vi "Main.vi"() -> ()   [LabVIEW 2017]
uses:
  <vilib>/Analysis/baseanly.llb/Mean (DBL).vi
  <vilib>/Analysis/NI_AALBase.lvlib
panel:
  in  "Save Raw Spectrometer Data":bool=TRUE
  out "Spectrometer Data":T1={[750.0, 800.0], "mean"=-22.554463094146342, array[2540 elements], array[2540 elements], "Color Temperatures"=[[-3182.0998200450113], [-4677.963743364752], [-7826.4943596651665]]}
  out "Voltage Average":dbl
  in  "Wait time (ms)":i32=250
  out "Motor Cluster":cluster{"Motor Relative":dbl[]}={"Motor Relative"=[0.0900112499774972, 0.0, 0.0, 0.0]}
  in  "WL2":dbl=800.0 format="%#_13g"
  in  "WL1":dbl=750.0 format="%#_13g"
  in  "Y axis":T2(ring)=enum."Spectrometer intensity"
  in  "Clear data":bool
  in  "Vi Selection":bool[](array[boolean])=[FALSE, TRUE, TRUE, TRUE, FALSE]
  in  "base path":path=path "E:/Materials Testing"
  in  "Filename":string="Run1"
  in  "stop":bool
  out "XY Graph":cluster{"magnitude":dbl[], dbl[]}(graph)
  in  "X axis":T3(ring)=enum."Spectrometer Wavelength"
  # "Power Meter"
  # "Spectrometer"
  # "Sensors"
  # "Motor"
  # "Keithley"
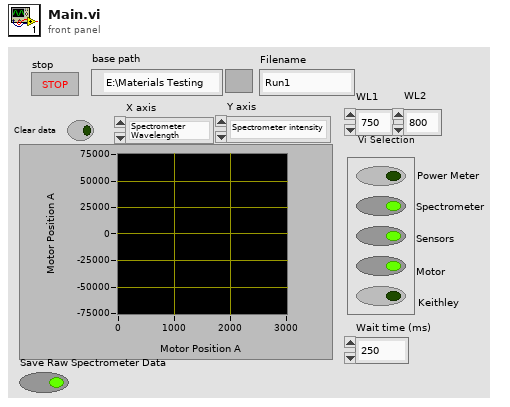
[diagram p1: front panel]
types:
  T1 = cluster{dbl[], "mean":dbl, dbl[], dbl[], "Color Temperatures":dbl[][]}
  T2 = enum16{"Motor Position A", "Motor Position B", "Motor Position C", "Motor Position D", "Spectrometer Region Avg.", "Keithley Voltage", "Spectrometer intensity", "Color Temp 2 -3", "Color Temp 1-3", "Color Temp 1-2"}
  T3 = enum16{"Time", "Motor Position A", "Motor Position B", "Motor Position C", "Motor Position D", "Spectrometer Wavelength"}
  T4 = enum16{"PowerMeter", "Spectrometer", "Sensors", "Motor", "Keithley"}
  T5 = enum32{"Invalid", "Standard", "Closed", "Hidden", "Minimized", "Maximized"}
  T6 = cluster{"output cluster 2":cluster{"Value:":dbl[], timestamp[], string[][]}, "output cluster 3":cluster{"Value:":dbl[], timestamp[], string[][]}}
  T7 = cluster{"Temperature Data":cluster{"Bandwidth":i32[], "Bandwidth labels":string[], "Color Temperatures":dbl[][], "Wavelength labels":string[], "seconds since 1Jan1904":timestamp}, "Vis Data":cluster{cluster{"visible wl array":dbl[], dbl[]}, cluster{"Vis or NIR":string, "Multiplexer Response":string, "Wavelength Difference Vis (nm)":dbl, "Vis Integration Time (ms)":u32, "Normalization path":path, "Vis background wave":cluster{dbl[], dbl[]}}}, "NIR Data":cluster{cluster{"NIR wl array":dbl[], dbl[]}, cluster{"Vis or NIR":string, "Multiplexer Response":string, "NIR Integration Time (ms)":u32, "Wavelength Difference NIR (nm) ":dbl, "Normalization path":path, "NIR background wave":cluster{dbl[], dbl[]}}}}
  T8 = cluster{dynamicdata, dynamicdata, dynamicdata, "Dynamic Data Type":dynamicdata}
  T9 = cluster{"Motor Relative":dbl[], "Motor absolute":dbl[], "Motor zero":dbl[], "Time between steps":dbl, "Conversion (steps/mm)":dbl[], "Distance  (mm)":dbl[], "run number":i32, "Number of steps":i32}
  T10 = cluster{"mean":dbl, "seconds since 1Jan1904":timestamp}
  T11 = enum32{"Bad", "Idle", "Run top level", "Running"}
  T12 = cluster{"VI out":refnum<vi>, "error out":errorcluster, refnum<vi>, enum16{"PowerMeter", "Spectrometer", "Sensors", "Motor", "Keithley"}, "Run Power meter":bool}
  T13 = enum16{"open", "open or create", "create or replace", "create", "open (read-only)"}
  T14 = cluster{"Bandwidth":i32[], "Bandwidth labels":string[], "Color Temperatures":dbl[][], "Wavelength labels":string[], "seconds since 1Jan1904":timestamp}
  T15 = cluster{cluster{"visible wl array":dbl[], dbl[]}, cluster{"Vis or NIR":string, "Multiplexer Response":string, "Wavelength Difference Vis (nm)":dbl, "Vis Integration Time (ms)":u32, "Normalization path":path, "Vis background wave":cluster{dbl[], dbl[]}}}
  T16 = cluster{cluster{"NIR wl array":dbl[], dbl[]}, cluster{"Vis or NIR":string, "Multiplexer Response":string, "NIR Integration Time (ms)":u32, "Wavelength Difference NIR (nm) ":dbl, "Normalization path":path, "NIR background wave":cluster{dbl[], dbl[]}}}
  T17 = cluster{"Vis or NIR":string, "Multiplexer Response":string, "NIR Integration Time (ms)":u32, "Wavelength Difference NIR (nm) ":dbl, "Normalization path":path, "NIR background wave":cluster{dbl[], dbl[]}}
  T18 = cluster{"Vis or NIR":string, "Multiplexer Response":string, "Wavelength Difference Vis (nm)":dbl, "Vis Integration Time (ms)":u32, "Normalization path":path, "Vis background wave":cluster{dbl[], dbl[]}}
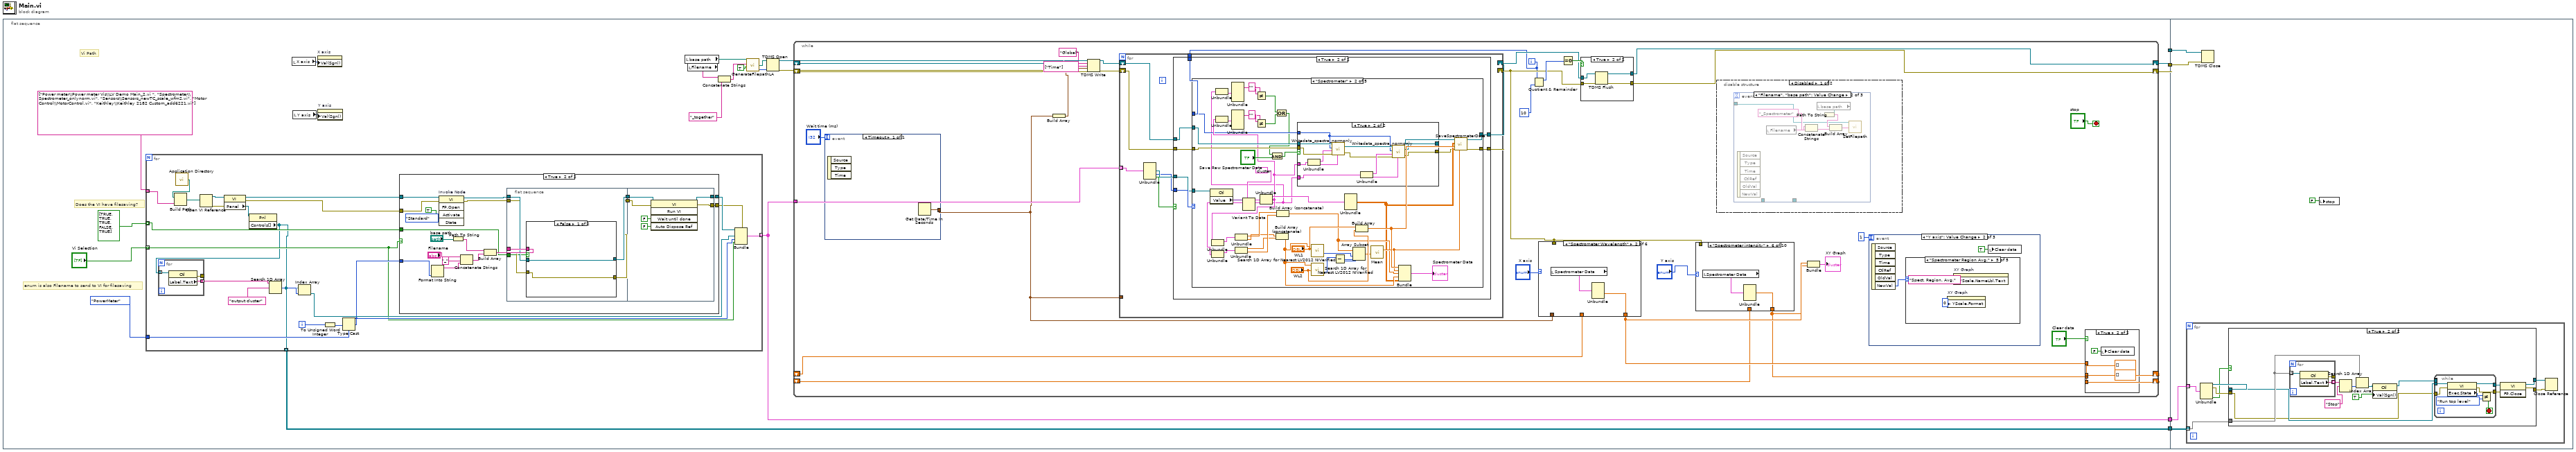
[diagram p0: block diagram]
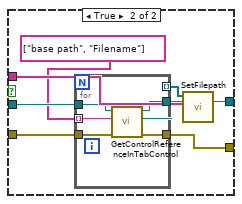
[diagram p3: hidden frame]
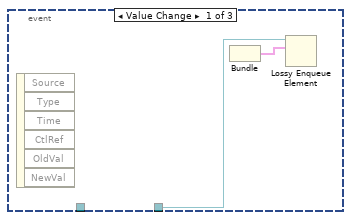
[diagram p5: hidden frame]
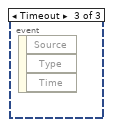
[diagram p6: hidden frame]
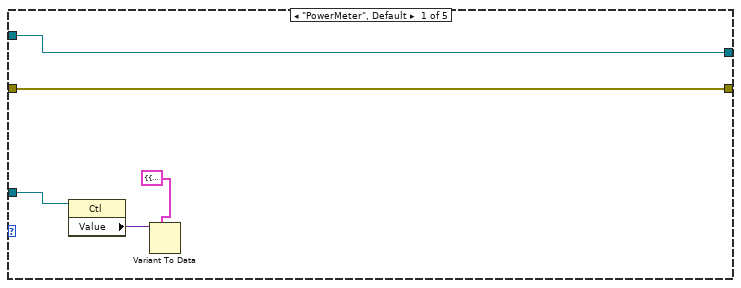
[diagram p9: hidden frame]
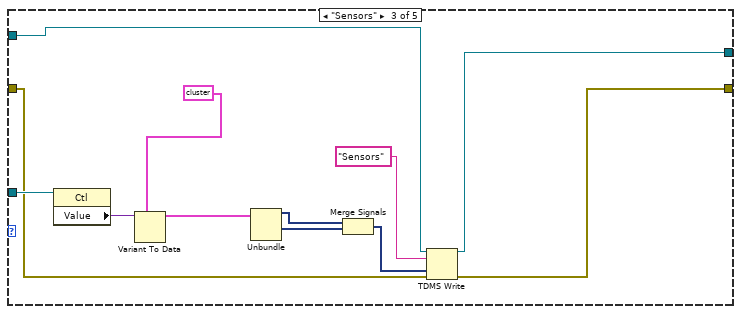
[diagram p11: hidden frame]
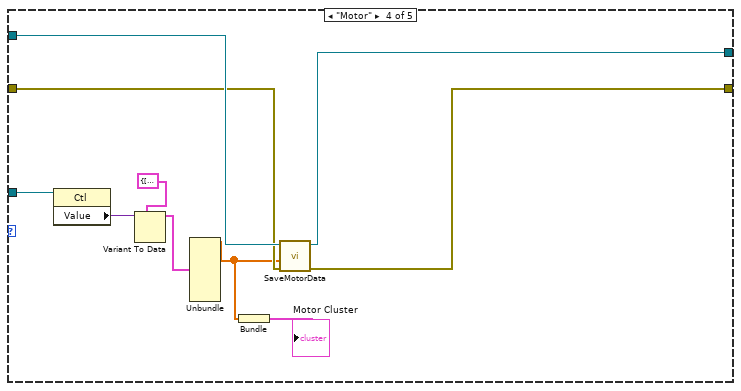
[diagram p12: hidden frame]
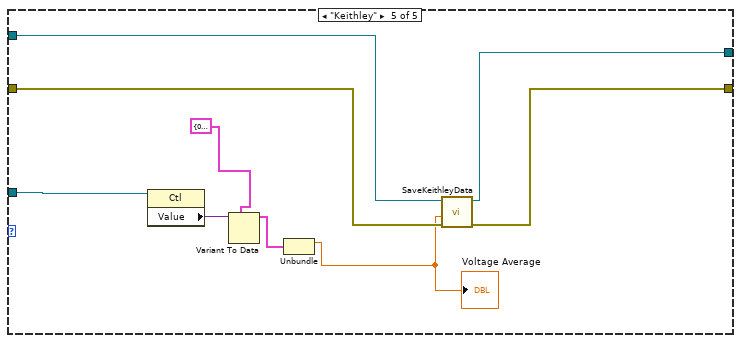
[diagram p13: hidden frame]
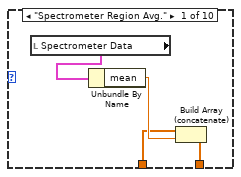
[diagram p15: hidden frame]
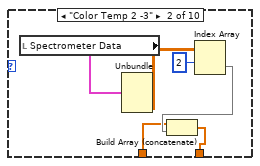
[diagram p16: hidden frame]
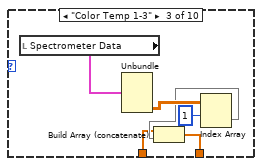
[diagram p17: hidden frame]
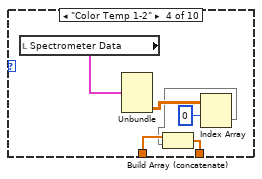
[diagram p18: hidden frame]
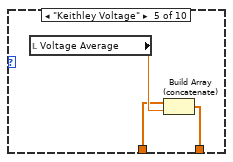
[diagram p19: hidden frame]
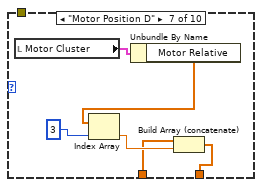
[diagram p20: hidden frame]
diagram:
  n1 = flat-sequence {
    tunnel: [w9] -> w4
    tunnel: [w10] -> w3
    tunnel: [w11] -> w2
    tunnel: [w7] -> w1
    tunnel: w4 -> [w370]
    tunnel: w3 -> [w369]
    tunnel: w2 -> [w368]
    tunnel: w1 -> [w367]
    frame #0 {
      # "Does the VI have filesaving?"
      # "enum is also Filename to send to VI for filesaving"
      # "Vi Path"
      n2 = for {
        tunnel: string[] ["Power meter\\Power meter Vis\\LV Demo Main_2.vi ", "Spectrometer\\Spectrometer_onlynorm.vi", "Sensors\\Sensors_newTC_scale_wfm2.vi", "Motor Control\\MotorControl.vi", "Keithley\\Keithley 2182 Custom_add6221.vi"] ("name or relative path") -> [w45] mode=indexing
        tunnel: bool[] [TRUE, TRUE, TRUE, FALSE, TRUE] ("Vi Selection 2") -> [w26] mode=indexing
        tunnel: T4."PowerMeter" -> [w44]
        tunnel: [w29] -> w11 mode=indexing
        tunnel: "Vi Selection" -> [w25] mode=indexing
        tunnel: [w24] -> w7 mode=indexing
        i -> [w43]
        n3 = call <vilib>:"Application Directory.vi"() -> ("Application Directory"=w38:path)
        n4 = Build Path(base path=w38, name or relative path=w45) -> (appended path=w34:path)
        n5 = Open VI Reference(vi path=w34) -> (vi reference=w36:refnum<vi>, error out=w37:errorcluster)  [unwired: 5 in]
        n6 = property class="VI"(reference=w36, error in=w37) -> (reference out=w41:refnum<vi>, error out=w39:errorcluster, "Panel"=w42:refnum<vi>)
        n7 = property class="Pnl"(reference=w42) -> ("Controls[]"=w24:refnum<vi>[])  [unwired: 1 in, 2 out]
        n8 = for {
          tunnel: w24 -> [w96] mode=indexing
          tunnel: [w95] -> w40 mode=indexing
          tunnel: [w94] -> _
          n9 = property class="Ctl"(reference=w96) -> (error out=w94:errorcluster, "Label.Text"=w95:string)  [unwired: 1 in, 1 out]
        }
        n10 = Search 1D Array(1D array=w40, element="output cluster") -> (index of element=w35:i32)  [unwired: 1 in]
        n11 = Index Array(array=w24, index=w35) -> (element=w28:refnum<vi>)
        n12 = To Unsigned Word Integer(number=w43) -> (unsigned 16bit integer=w30:u16)
        n13 = Type Cast(type=w44, x=w30) -> (*(type *) &x=w27:T4)
        n14 = case shown="True" w25 {
          tunnel: [w47 w59] -> w32
          tunnel: [w46 w58] -> w31
          tunnel: w41 -> [w47 w53]
          tunnel: w39 -> [w46 w52]
          tunnel: w27 -> [_ w49]
          tunnel: w26 -> [_ w48]
          frame False {
          }
          frame True {
            n15 = Format Into String(w49) -> (resulting string=w56:string)  [unwired: 3 in, 1 out]
            n16 = invoke on="Invoke Node" class="VI" method="FP.Open"(reference=w53, error in=w52, "Activate"=TRUE ("Activate?"), "State"=T5."Standard") -> (reference out=w51:refnum<vi>, error out=w50:errorcluster)  [unwired: 1 in, 3 out]
            n17 = Path To String(path="base path") -> (string=w62:string)
            n18 = Concatenate Strings("Filename", "_" ("string"), w56) -> (w63:string)
            n19 = Build Array(w62, w63) -> (w64:string[])
            n20 = flat-sequence {
              tunnel: w50 -> [w70]
              tunnel: w64 -> [w72]
              tunnel: w51 -> [w71]
              tunnel: [w69] -> w66
              tunnel: [w68] -> w65
              tunnel: w48 -> [w67]
              tunnel: w66 -> [w91]
              tunnel: w65 -> [w89]
              tunnel: [w90] -> w59
              tunnel: [w88] -> w58
              frame #0 {
                n21 = case shown="False" w67 {
                  tunnel: w72 -> [_ w81]
                  tunnel: w71 -> [w74 w79]
                  tunnel: w70 -> [w73 w78]
                  tunnel: [w74 w76] -> w69
                  tunnel: [w73 w75] -> w68
                  frame False {
                  }
                  frame True {
                    n22 = for {
                      tunnel: string[] ["base path", "Filename"] -> [w87] mode=indexing
                      tunnel: w79 -> [w86]
                      tunnel: w78 -> [w85]
                      tunnel: [w84] -> w76
                      tunnel: [w83] -> w75
                      tunnel: [w82] -> w80 mode=indexing
                      n23 = call "GetControlReferenceInTabControl.vi"("error in (no error)"=w85, "Control Name"=w87, "VI in"=w86) -> ("error out"=w83:errorcluster, "Ctl Refnum"=w82:refnum<vi>, "VI out"=w84:refnum<vi>)  [unwired: 6 in]
                    }
                    n24 = call "SetFilepath.vi"("Array 2"=w81, "Array"=w80) -> ()  [unwired: 10 in]
                  }
                }
              }
              frame #1 {
                n25 = invoke class="VI" method="Run VI"(reference=w91, error in=w89, "Wait until done"=FALSE ("Wait Until Done"), "Auto Dispose Ref"=FALSE ("Auto Dispose Reference")) -> (reference out=w90:refnum<vi>, error out=w88:errorcluster)  [unwired: 1 in, 3 out]
              }
            }
          }
        }
        n26 = Bundle("VI out"=w32, "error out"=w31, w28, w27, "Run Power meter"=w25) -> (w29:T12)  [unwired: 1 in]
      }
      n27 = local read "X axis"() -> (w6:T3)
      n28 = local read "Y axis"() -> (w5:T2)
      n29 = property on="X axis" class="Enum (strict)"("Val(Sgnl)"=w6) -> ()  [unwired: 2 in, 2 out]
      n30 = property on="Y axis" class="Enum (strict)"("Val(Sgnl)"=w5) -> ()  [unwired: 2 in, 2 out]
      n31 = local read "base path"() -> (w21:path)
      n32 = local read "Filename"() -> (w17:string)
      n33 = Concatenate Strings(w17, "_together" ("string")) -> (w15:string)
      n34 = call "GenerateFilepathLA.vi"("Auto Date folder"=TRUE, "Filename"=w15, "base path"=w21) -> ("operation (0:open)"=w22:T13, "file path"=w20:path)  [unwired: 1 in, 1 out]
      n35 = TDMS Open(10:w22, 11:w20) -> (0:w19:errorcluster, 3:w18:refnum<k34>)  [unwired: 5 in]
      n36 = while {
        shift-right: [w106] -> w10
        shift-left: w18 -> [w115]
        shift-right: [w105] -> w9
        shift-left: w19 -> [w116]
        tunnel: w11 -> [w119]
        shift-right: [w108] -> _
        shift-left: _ -> [w100]
        shift-right: [w109] -> _
        shift-left: _ -> [w98]
        i -> [w97]
        stop <- "stop" stop-if-true
        n37 = event shown="[0] Timeout" {
          selector: _ -> [_]
          dyn-events: _ -> [_]
          timeout: "Wait time (ms)" -> [_]
          tunnel: [w127] -> w103
          event Timeout {
            n38 = event-data() -> ()  [unwired: 1 in, 3 out]
            n39 = Get Date/Time In Seconds() -> (seconds since 1Jan1904=w127:timestamp)
          }
        }
        n40 = Build Array(w103) -> (w114:timestamp[])
        n41 = TDMS Write(0:w115, 5:"Global" ("group name in (Untitled)"), 7:string[] ["Time"] ("channel name(s) in (Untitled)"), 9:w114, 11:w116) -> (4:w111:refnum<k34>, 15:w110:errorcluster)  [unwired: 1 in, 2 out]
        n42 = for {
          tunnel: w119 -> [w152] mode=indexing
          shift-right: [w149] -> w118
          shift-left: w111 -> [w151]
          shift-right: [w148] -> w104
          shift-left: w110 -> [w150]
          tunnel: w103 -> [_]
          tunnel: w97 -> [w144]
          n43 = Unbundle(w152) -> (w147:refnum<vi>, w146:T4, "Run Power meter"=w145:bool)  [unwired: 2 out]
          n44 = case shown="True" w145 {
            tunnel: w146 -> [_ w161]
            tunnel: w147 -> [_ w160]
            tunnel: w151 -> [w154 w159]
            tunnel: w150 -> [w153 w158]
            tunnel: [w154 w157] -> w149
            tunnel: [w153 w156] -> w148
            tunnel: w144 -> [_ w155]
            frame False {
            }
            frame True {
              n45 = case shown="\"Spectrometer\"" w161 {
                tunnel: w160 -> [w165 w209 w236 w246 w253]
                tunnel: w159 -> [w163 w182 w233 w242 w252]
                tunnel: w158 -> [w162 w181 w232 w240 w251]
                tunnel: [w163 w201 w229 w241 w250] -> w157
                tunnel: [w162 w200 w231 w239 w249] -> w156
                tunnel: w155 -> [_ w174 _ _ _]
                frame "PowerMeter", Default {
                  n46 = property class="Ctl"(reference=w165) -> ("Value"=w166:variant)  [unwired: 1 in, 2 out]
                  n47 = Variant To Data(type=T6 {"output cluster 2"={"Value:"=[], [], []}, "output cluster 3"={"Value:"=[], [], []}} ("Power meter Cluster 2"), Variant=w166) -> ()  [unwired: 1 in, 2 out]
                }
                frame "Spectrometer" {
                  n48 = property class="Ctl"(reference=w209) -> ("Value"=w208:variant)  [unwired: 1 in, 2 out]
                  n49 = Variant To Data(type=T7 {"Temperature Data"={"Bandwidth"=[10, 10, 10], "Bandwidth labels"=["Bandwidth 1-2", "Bandwidth 2-3", "Bandwidth 1-3"], "Color Temperatures"=[[879.3311636229715], [-21903.619530261916], [-1063.75969736004]], "Wavelength labels"=["Temp1050-1120", "Temp1050-1230", "Temp1120-1230"], "seconds since 1Jan1904"=timestamp(3594756427.269044 s since 1904-01-01)}, "Vis Data"={{"visible wl array"=array[512 elements], array[512 elements]}, {"Vis or NIR"="NIR", "Multiplexer Response"="-1", "Wavelength Difference Vis (nm)"=50.0, "Vis Integration Time (ms)"=100, "Normalization path"=path "E:/Materials Testing/Calibration/2017-11-09/Multiplexter.tdms", "Vis background wave"={array[512 elements], array[512 elements]}}}, "NIR Data"={{"NIR wl array"=array[2028 elements], array[2028 elements]}, {"Vis or NIR"="Visible", "Multiplexer Response"="-1", "NIR Integration Time (ms)"=100, "Wavelength Difference NIR (nm) "=100.0, "Normalization path"=path "E:/Materials Testing/Calibration/2017-11-09/Multiplexter.tdms", "NIR background wave"={array[2028 elements], array[2028 elements]}}}} ("output cluster"), Variant=w208) -> (data=w197:T7)  [unwired: 1 in, 1 out]
                  n50 = Unbundle(w197) -> ("Temperature Data"=w183:T14, "Vis Data"=w175:T15, "NIR Data"=w170:T16)
                  n51 = Unbundle(w175) -> (w189:cluster{"visible wl array":dbl[], dbl[]})  [unwired: 1 out]
                  n52 = Unbundle(w170) -> (w188:cluster{"NIR wl array":dbl[], dbl[]})  [unwired: 1 out]
                  n53 = Unbundle(w170) -> (w172:T17)  [unwired: 1 out]
                  n54 = Unbundle(w175) -> (w177:T18)  [unwired: 1 out]
                  n55 = Unbundle(w172) -> ("Multiplexer Response"=w173:string)  [unwired: 5 out]
                  n56 = Unbundle(w177) -> ("Multiplexer Response"=w176:string)  [unwired: 5 out]
                  n57 = Unbundle(w188) -> ("NIR wl array"=w184:dbl[], w186:dbl[])
                  n58 = Unbundle(w189) -> ("visible wl array"=w185:dbl[], w187:dbl[])
                  n59 = Not Equal?(x="", y=w173) -> (x != y?=w169:bool)
                  n60 = Not Equal?(x="", y=w176) -> (x != y?=w168:bool)
                  n61 = Or(x=w169, y=w168) -> (x .or. y?=w167:bool)
                  n62 = And(x=w167, y="Save Raw Spectrometer Data") -> (x .and. y?=w178:bool)
                  n63 = Build Array (concatenate)(w185, w184) -> (w196:dbl[])
                  n64 = Build Array (concatenate)(w187, w186) -> (w195:dbl[])
                  n65 = case shown="True" w178 {
                    tunnel: [w211 w214] -> w180
                    tunnel: w182 -> [w211 w224]
                    tunnel: [w210 w213] -> w179
                    tunnel: w181 -> [w210 w223]
                    tunnel: w175 -> [_ w222]
                    tunnel: w170 -> [_ w219]
                    tunnel: w174 -> [_ w212]
                    frame False {
                    }
                    frame True {
                      n66 = Unbundle(w222) -> (w221:cluster{"visible wl array":dbl[], dbl[]}, w220:T18)
                      n67 = call "Writedata_spectra_normonly.vi"("tdms file in"=w224, "Aquisition number"=w212, "Norm Visible Intensity"=w221, "tdms error in"=w223, "Params"=w220) -> ("tdms file out"=w216:refnum<k34>, "tdms error out"=w215:errorcluster)
                      n68 = Unbundle(w219) -> (w218:cluster{"NIR wl array":dbl[], dbl[]}, w217:T17)
                      n69 = call "Writedata_spectra_normonly.vi"("tdms file in"=w216, "Aquisition number"=w212, "Norm Visible Intensity"=w218, "tdms error in"=w215, "Params"=w217) -> ("tdms file out"=w214:refnum<k34>, "tdms error out"=w213:errorcluster)
                    }
                  }
                  n70 = call "Search 1D Array for Nearest LV2012 NIVerified.vi"("desired element"="WL1", "1D Array"=w196) -> ("closest index"=w202:i32)  [unwired: 8 in, 1 out]
                  n71 = call "Search 1D Array for Nearest LV2012 NIVerified.vi"("desired element"="WL2", "1D Array"=w196) -> ("closest index"=w203:i32)  [unwired: 8 in, 1 out]
                  n72 = Subtract(x=w203, y=w202) -> (x-y=w204:i32)
                  n73 = Unbundle(w183) -> ("Color Temperatures"=w191:dbl[][])  [unwired: 4 out]
                  n74 = Array Subset(array=w195, index=w202, length=w204) -> (w205:dbl[])
                  n75 = Build Array("WL1", "WL2") -> (w199:dbl[])
                  n76 = call-poly <vilib>:"Mean.vi"("X"=w205) -> ("mean"=w198:dbl)  [unwired: 1 out]
                  n77 = Bundle(w199, "mean"=w198, w195, w196, "Color Temperatures"=w191) -> (→"Spectrometer Data":T1)  [unwired: 1 in]
                  n78 = call "SaveSpectrometerData.vi"("Average"=w198, "error in (no error)"=w179, "Wavelengths"=w199, "Color Temperatures"=w191, "Refnum in"=w180) -> ("error out"=w200:errorcluster, "Refnum out"=w201:refnum<k34>)  [unwired: 5 in]
                }
                frame "Sensors" {
                  n79 = property class="Ctl"(reference=w236) -> ("Value"=w235:variant)  [unwired: 1 in, 2 out]
                  n80 = Variant To Data(type=T8 {[], [], [], "Dynamic Data Type"=[]} ("output cluster"), Variant=w235) -> (data=w234:T8)  [unwired: 1 in, 1 out]
                  n81 = Unbundle(w234) -> (w228:dynamicdata, w227:dynamicdata)  [unwired: 2 out]
                  n82 = Merge Signals(w228, w227) -> (w226:dynamicdata)
                  n83 = TDMS Write(0:w233, 5:"Sensors" ("group name in (Untitled)"), 9:w226, 11:w232) -> (4:w229:refnum<k34>, 15:w231:errorcluster)  [unwired: 2 in, 2 out]
                }
                frame "Motor" {
                  n84 = property class="Ctl"(reference=w246) -> ("Value"=w245:variant)  [unwired: 1 in, 2 out]
                  n85 = Variant To Data(type=T9 {"Motor Relative"=[], "Motor absolute"=[], "Motor zero"=[], "Time between steps"=0.0, "Conversion (steps/mm)"=[], "Distance  (mm)"=[], "run number"=0, "Number of steps"=0} ("output cluster 2"), Variant=w245) -> (data=w244:T9)  [unwired: 1 in, 1 out]
                  n86 = Unbundle(w244) -> ("Motor Relative"=w237:dbl[])  [unwired: 7 out]
                  n87 = Bundle("Motor Relative"=w237) -> (→"Motor Cluster":cluster{"Motor Relative":dbl[]})  [unwired: 1 in]
                  n88 = call "SaveMotorData.vi"("error in (no error)"=w240, "Motor Relative"=w237, "Refnum in"=w242) -> ("error out"=w239:errorcluster, "Refnum out"=w241:refnum<k34>)  [unwired: 7 in]
                }
                frame "Keithley" {
                  n89 = property class="Ctl"(reference=w253) -> ("Value"=w255:variant)  [unwired: 1 in, 2 out]
                  n90 = Variant To Data(type=T10 {"mean"=0.0, "seconds since 1Jan1904"=timestamp(0 s since 1904-01-01)} ("output cluster 2"), Variant=w255) -> (data=w254:T10)  [unwired: 1 in, 1 out]
                  n91 = Unbundle(w254) -> ("mean"=w247:dbl)  [unwired: 1 out]
                  "Voltage Average" <- w247
                  n92 = call "SaveKeithleyData.vi"("error in (no error)"=w251, "Voltage average"=w247, "Refnum in"=w252) -> ("error out"=w249:errorcluster, "Refnum out"=w250:refnum<k34>)  [unwired: 7 in]
                }
              }
            }
          }
        }
        n93 = Quotient & Remainder(x=w97, y=10) -> (x-y*floor(x/y)=w120:i32)  [unwired: 1 out]
        n94 = case shown="\"Spectrometer Wavelength\"" "X axis" {
          tunnel: w103 -> [w316 _ _ _ _ _]
          tunnel: w104 -> [_ _ _ _ _ _]
          tunnel: [w314 w317 w319 w326 w332 w337] -> w101
          tunnel: w100 -> [w313 _ w320 w325 w331 w338]
          frame "Time" {
            n95 = To Double Precision Float(number=w316) -> (double precision float=w315:dbl)
            n96 = Build Array (concatenate)(w313, w315) -> (w314:dbl[])
          }
          frame "Spectrometer Wavelength" {
            n97 = local read "Spectrometer Data"() -> (w318:T1)
            n98 = Unbundle(w318) -> (w317:dbl[])  [unwired: 4 out]
          }
          frame "Motor Position A" {
            n99 = local read "Motor Cluster"() -> (w324:cluster{"Motor Relative":dbl[]})
            n100 = Unbundle By Name(w324) -> ("Motor Relative"=w323:dbl[])
            n101 = Index Array(array=w323, index=0 ("disabled index (col)")) -> (element=w321:dbl)
            n102 = Build Array (concatenate)(w320, w321) -> (w319:dbl[])
          }
          frame "Motor Position B" {
            n103 = local read "Motor Cluster"() -> (w330:cluster{"Motor Relative":dbl[]})
            n104 = Unbundle By Name(w330) -> ("Motor Relative"=w329:dbl[])
            n105 = Index Array(array=w329, index=1 ("disabled index (col)")) -> (element=w327:dbl)
            n106 = Build Array (concatenate)(w325, w327) -> (w326:dbl[])
          }
          frame "Motor Position C" {
            n107 = local read "Motor Cluster"() -> (w336:cluster{"Motor Relative":dbl[]})
            n108 = Unbundle By Name(w336) -> ("Motor Relative"=w335:dbl[])
            n109 = Index Array(array=w335, index=2 ("disabled index (col)")) -> (element=w333:dbl)
            n110 = Build Array (concatenate)(w331, w333) -> (w332:dbl[])
          }
          frame "Motor Position D" {
            n111 = local read "Motor Cluster"() -> (w342:cluster{"Motor Relative":dbl[]})
            n112 = Unbundle By Name(w342) -> ("Motor Relative"=w341:dbl[])
            n113 = Index Array(array=w341, index=3 ("disabled index (col)")) -> (element=w339:dbl)
            n114 = Build Array (concatenate)(w338, w339) -> (w337:dbl[])
          }
        }
        n115 = Equal To 0?(x=w120) -> (x = 0?=w121:bool)
        n116 = case shown="True" w121 {
          tunnel: [w256 w261] -> w106
          tunnel: [w257 w260] -> w105
          tunnel: w104 -> [w257 w259]
          tunnel: w118 -> [w256 w258]
          frame False {
          }
          frame True {
            n117 = TDMS Flush(4:w259, 7:w258) -> (0:w260:errorcluster, 3:w261:refnum<k34>)
          }
        }
        n118 = case shown="\"Spectrometer intensity\"" "Y axis" {
          tunnel: w104 -> [_ _ _ _ _ _ _ _ _ _]
          tunnel: [w263 w268 w274 w278 w284 w287 w289 w295 w301 w307] -> w99
          tunnel: w98 -> [w262 w266 w272 w280 w285 _ w290 w296 w302 w308]
          frame "Spectrometer Region Avg." {
            n119 = local read "Spectrometer Data"() -> (w265:T1)
            n120 = Unbundle By Name(w265) -> ("mean"=w264:dbl)
            n121 = Build Array (concatenate)(w262, w264) -> (w263:dbl[])
          }
          frame "Color Temp 2 -3" {
            n122 = local read "Spectrometer Data"() -> (w271:T1)
            n123 = Unbundle(w271) -> ("Color Temperatures"=w270:dbl[][])  [unwired: 4 out]
            n124 = Index Array(array=w270, index (row)=2) -> (element=w267:dbl[])  [unwired: 1 in]
            n125 = Build Array (concatenate)(w266, w267) -> (w268:dbl[])
          }
          frame "Color Temp 1-3" {
            n126 = local read "Spectrometer Data"() -> (w277:T1)
            n127 = Unbundle(w277) -> ("Color Temperatures"=w276:dbl[][])  [unwired: 4 out]
            n128 = Index Array(array=w276, index (row)=1) -> (element=w273:dbl[])  [unwired: 1 in]
            n129 = Build Array (concatenate)(w272, w273) -> (w274:dbl[])
          }
          frame "Color Temp 1-2" {
            n130 = local read "Spectrometer Data"() -> (w283:T1)
            n131 = Unbundle(w283) -> ("Color Temperatures"=w282:dbl[][])  [unwired: 4 out]
            n132 = Index Array(array=w282, index (row)=0) -> (element=w279:dbl[])  [unwired: 1 in]
            n133 = Build Array (concatenate)(w280, w279) -> (w278:dbl[])
          }
          frame "Keithley Voltage" {
            n134 = local read "Voltage Average"() -> (w286:dbl)
            n135 = Build Array (concatenate)(w285, w286) -> (w284:dbl[])
          }
          frame "Spectrometer intensity" {
            n136 = local read "Spectrometer Data"() -> (w288:T1)
            n137 = Unbundle(w288) -> (w287:dbl[])  [unwired: 4 out]
          }
          frame "Motor Position D" {
            n138 = local read "Motor Cluster"() -> (w292:cluster{"Motor Relative":dbl[]})
            n139 = Unbundle By Name(w292) -> ("Motor Relative"=w293:dbl[])
            n140 = Index Array(array=w293, index=3 ("disabled index (col)")) -> (element=w291:dbl)
            n141 = Build Array (concatenate)(w290, w291) -> (w289:dbl[])
          }
          frame "Motor Position C" {
            n142 = local read "Motor Cluster"() -> (w298:cluster{"Motor Relative":dbl[]})
            n143 = Unbundle By Name(w298) -> ("Motor Relative"=w299:dbl[])
            n144 = Index Array(array=w299, index=2 ("disabled index (col)")) -> (element=w297:dbl)
            n145 = Build Array (concatenate)(w296, w297) -> (w295:dbl[])
          }
          frame "Motor Position B" {
            n146 = local read "Motor Cluster"() -> (w304:cluster{"Motor Relative":dbl[]})
            n147 = Unbundle By Name(w304) -> ("Motor Relative"=w305:dbl[])
            n148 = Index Array(array=w305, index=1 ("disabled index (col)")) -> (element=w303:dbl)
            n149 = Build Array (concatenate)(w302, w303) -> (w301:dbl[])
          }
          frame "Motor Position A" {
            n150 = local read "Motor Cluster"() -> (w310:cluster{"Motor Relative":dbl[]})
            n151 = Unbundle By Name(w310) -> ("Motor Relative"=w311:dbl[])
            n152 = Index Array(array=w311, index=0 ("disabled index (col)")) -> (element=w309:dbl)
            n153 = Build Array (concatenate)(w308, w309) -> (w307:dbl[])
          }
        }
        n154 = disable-structure shown="Disabled" {
          frame Disabled {
            n155 = event shown="[1] \"Filename\", \"base path\": Value Change" {
              selector: _ -> [_ _ _]
              dyn-events: _ -> [_ _ _]
              timeout: _ -> [_ _ _]
              tunnel: _ -> [_ _ _]
              tunnel: _ -> [_ w137 _]
              tunnel: _ -> [w135 _ _]
              event Value Change {
                n156 = event-data() -> ("NewVal"=w136:variant)  [unwired: 1 in, 5 out]
                n157 = Bundle() -> (w134:cluster{void, void}, w133)  [unwired: 2 in]
                n158 = Lossy Enqueue Element(queue=w135, element=w134) -> ()  [unwired: 1 in, 4 out]
              }
              event "Filename", "base path": Value Change {
                n159 = event-data() -> ()  [unwired: 1 in, 6 out]
                n160 = local read "Filename"() -> (w140:string)
                n161 = Concatenate Strings(w140, "_Spectrometer" ("string")) -> (w141:string)
                n162 = local read "base path"() -> (w139:path)
                n163 = Path To String(path=w139) -> (string=w142:string)
                n164 = Build Array(w142, w141) -> (w138:string[])
                n165 = call "SetFilepath.vi"("Array 2"=w138, "Array"=w137) -> ()  [unwired: 10 in]
              }
              event Timeout {
                n166 = event-data() -> ()  [unwired: 1 in, 3 out]
              }
            }
          }
          frame Enabled {
          }
        }
        n167 = Bundle(w101, w99) -> (→"XY Graph":cluster{dbl[], dbl[]})  [unwired: 1 in]
        n168 = event shown="[1] \"Y axis\": Value Change" {
          selector: _ -> [_ _ _]
          dyn-events: _ -> [_ _ _]
          timeout: 1 -> [_ _ _]
          event "X axis": Value Change {
            n169 = event-data() -> ("NewVal"=w344:T3)  [unwired: 1 in, 5 out]
            n170 = case shown="\"Time\"" w344 {
              frame "Time" {
                n171 = property on="XY Graph" class="XYGraph (strict)"("XScale.Format"=u8 7 ("Y Scale.Display Format:Format")) -> ()  [unwired: 2 in, 2 out]
                n172 = property on="XY Graph" class="XYGraph (strict)"("XScale.NameLbl.Text"="Time" ("X Scale.Name Label.Text")) -> ()  [unwired: 2 in, 2 out]
              }
              frame "Motor Position A", Default {
                n173 = property on="XY Graph" class="XYGraph (strict)"("XScale.NameLbl.Text"="Motor Position A" ("X Scale.Name Label.Text")) -> ()  [unwired: 2 in, 2 out]
                n174 = property on="XY Graph" class="XYGraph (strict)"("XScale.Format"=u8 0 ("Y Scale.Display Format:Format")) -> ()  [unwired: 2 in, 2 out]
              }
              frame "Motor Position B" {
                n175 = property on="XY Graph" class="XYGraph (strict)"("XScale.NameLbl.Text"="Motor Position B" ("X Scale.Name Label.Text")) -> ()  [unwired: 2 in, 2 out]
                n176 = property on="XY Graph" class="XYGraph (strict)"("XScale.Format"=u8 0 ("Y Scale.Display Format:Format")) -> ()  [unwired: 2 in, 2 out]
              }
              frame "Motor Position C" {
                n177 = property on="XY Graph" class="XYGraph (strict)"("XScale.NameLbl.Text"="Motor Position C" ("X Scale.Name Label.Text")) -> ()  [unwired: 2 in, 2 out]
                n178 = property on="XY Graph" class="XYGraph (strict)"("XScale.Format"=u8 0 ("Y Scale.Display Format:Format")) -> ()  [unwired: 2 in, 2 out]
              }
              frame "Motor Position D" {
                n179 = property on="XY Graph" class="XYGraph (strict)"("XScale.NameLbl.Text"="Motor Position D" ("X Scale.Name Label.Text")) -> ()  [unwired: 2 in, 2 out]
                n180 = property on="XY Graph" class="XYGraph (strict)"("XScale.Format"=u8 0 ("Y Scale.Display Format:Format")) -> ()  [unwired: 2 in, 2 out]
              }
            }
            n181 = local write "Clear data"(TRUE ("Clear data")) -> ()
          }
          event "Y axis": Value Change {
            n182 = event-data() -> ("NewVal"=w356:T2)  [unwired: 1 in, 5 out]
            n183 = case shown="\"Spectrometer Region Avg.\"" w356 {
              frame "Motor Position A", Default {
                n184 = property on="XY Graph" class="XYGraph (strict)"("YScale.Format"=u8 0 ("Y Scale.Display Format:Format")) -> ()  [unwired: 2 in, 2 out]
                n185 = property on="XY Graph" class="XYGraph (strict)"("YScale.NameLbl.Text"="Motor Position A" ("X Scale.Name Label.Text")) -> ()  [unwired: 2 in, 2 out]
              }
              frame "Motor Position B" {
                n186 = property on="XY Graph" class="XYGraph (strict)"("YScale.Format"=u8 0 ("Y Scale.Display Format:Format")) -> ()  [unwired: 2 in, 2 out]
                n187 = property on="XY Graph" class="XYGraph (strict)"("YScale.NameLbl.Text"="Motor Position B" ("X Scale.Name Label.Text")) -> ()  [unwired: 2 in, 2 out]
              }
              frame "Motor Position C" {
                n188 = property on="XY Graph" class="XYGraph (strict)"("YScale.Format"=u8 0 ("Y Scale.Display Format:Format")) -> ()  [unwired: 2 in, 2 out]
                n189 = property on="XY Graph" class="XYGraph (strict)"("YScale.NameLbl.Text"="Motor Position C" ("X Scale.Name Label.Text")) -> ()  [unwired: 2 in, 2 out]
              }
              frame "Motor Position D" {
                n190 = property on="XY Graph" class="XYGraph (strict)"("YScale.Format"=u8 0 ("Y Scale.Display Format:Format")) -> ()  [unwired: 2 in, 2 out]
                n191 = property on="XY Graph" class="XYGraph (strict)"("YScale.NameLbl.Text"="Motor Position D" ("X Scale.Name Label.Text")) -> ()  [unwired: 2 in, 2 out]
              }
              frame "Spectrometer Region Avg." {
                n192 = property on="XY Graph" class="XYGraph (strict)"("YScale.Format"=u8 0 ("Y Scale.Display Format:Format")) -> ()  [unwired: 2 in, 2 out]
                n193 = property on="XY Graph" class="XYGraph (strict)"("YScale.NameLbl.Text"="Spect. Region. Avg." ("X Scale.Name Label.Text")) -> ()  [unwired: 2 in, 2 out]
              }
            }
            n194 = local write "Clear data"(TRUE ("Clear data")) -> ()
          }
          event Timeout {
            n195 = event-data() -> ()  [unwired: 1 in, 3 out]
          }
        }
        n196 = case shown="True" "Clear data" {
          tunnel: w101 -> [w128 _]
          tunnel: w99 -> [w129 _]
          tunnel: [w129 dbl[] []] -> w109
          tunnel: [w128 dbl[] []] -> w108
          frame False {
          }
          frame True {
            n197 = local write "Clear data"(FALSE ("Clear data")) -> ()
          }
        }
      }
    }
    frame #1 {
      n198 = for {
        tunnel: w368 -> [w377] mode=indexing
        tunnel: w367 -> [w372] mode=indexing
        n199 = Unbundle(w377) -> ("VI out"=w376:refnum<vi>, "error out"=w375:errorcluster, "Run Power meter"=w373:bool)  [unwired: 2 out]
        n200 = case shown="True" w373 {
          tunnel: [w380 w392] -> w378
          tunnel: w376 -> [w380 w383]
          tunnel: w375 -> [w379 w382]
          tunnel: [w379 w391] -> w374
          tunnel: w372 -> [_ w385]
          frame False {
          }
          frame True {
            n201 = for {
              tunnel: w385 -> [w396] mode=indexing
              tunnel: [w395] -> w388 mode=indexing
              tunnel: [w394] -> _
              n202 = property class="Ctl"(reference=w396) -> (error out=w394:errorcluster, "Label.Text"=w395:string)  [unwired: 1 in, 1 out]
            }
            n203 = Search 1D Array(1D array=w388, element="Stop") -> (index of element=w387:i32)  [unwired: 1 in]
            n204 = Index Array(array=w385, index=w387) -> (element=w389:refnum<vi>)
            n205 = property class="Ctl"(reference=w389, "Val(Sgnl)"=TRUE) -> (reference out=w381:refnum<vi>)  [unwired: 1 in, 1 out]
            n206 = while {
              tunnel: w383 -> [w404]
              tunnel: [w403] -> w393
              tunnel: w382 -> [w399]
              tunnel: [w398] -> w390
              tunnel: [w397] -> _
              tunnel: w381 -> [w397]
              stop <- w402 stop-if-true
              n207 = property class="VI"(reference=w404, error in=w399) -> (reference out=w403:refnum<vi>, error out=w398:errorcluster, "Exec.State"=w401:T11)
              n208 = Not Equal?(x=w401, y=T11."Run top level" ("Execution:State 2")) -> (x != y?=w402:bool)
            }
            n209 = invoke class="VI" method="FP.Close"(reference=w393, error in=w390) -> (reference out=w392:refnum<vi>, error out=w391:errorcluster)  [unwired: 1 in, 1 out]
          }
        }
        n210 = Close Reference(reference=w378, error in (no error)=w374) -> ()  [unwired: 1 out]
      }
      n211 = TDMS Close(8:w370, 11:w369) -> ()  [unwired: 2 out]
      n212 = local write "stop"(FALSE ("stop")) -> ()
    }
  }
